vi "testVisa.vi"() -> ()   [LabVIEW 2026]
uses:
  <userlib>/Sensor.ctl
  <vilib>/Instr/_visa.llb/VISA Configure Serial Port (Instr).vi
panel:
  out "Waveform Chart":dbl(graph)
  out "Waveform Graph":waveform(dbl)(graph)
  in  "stop":bool
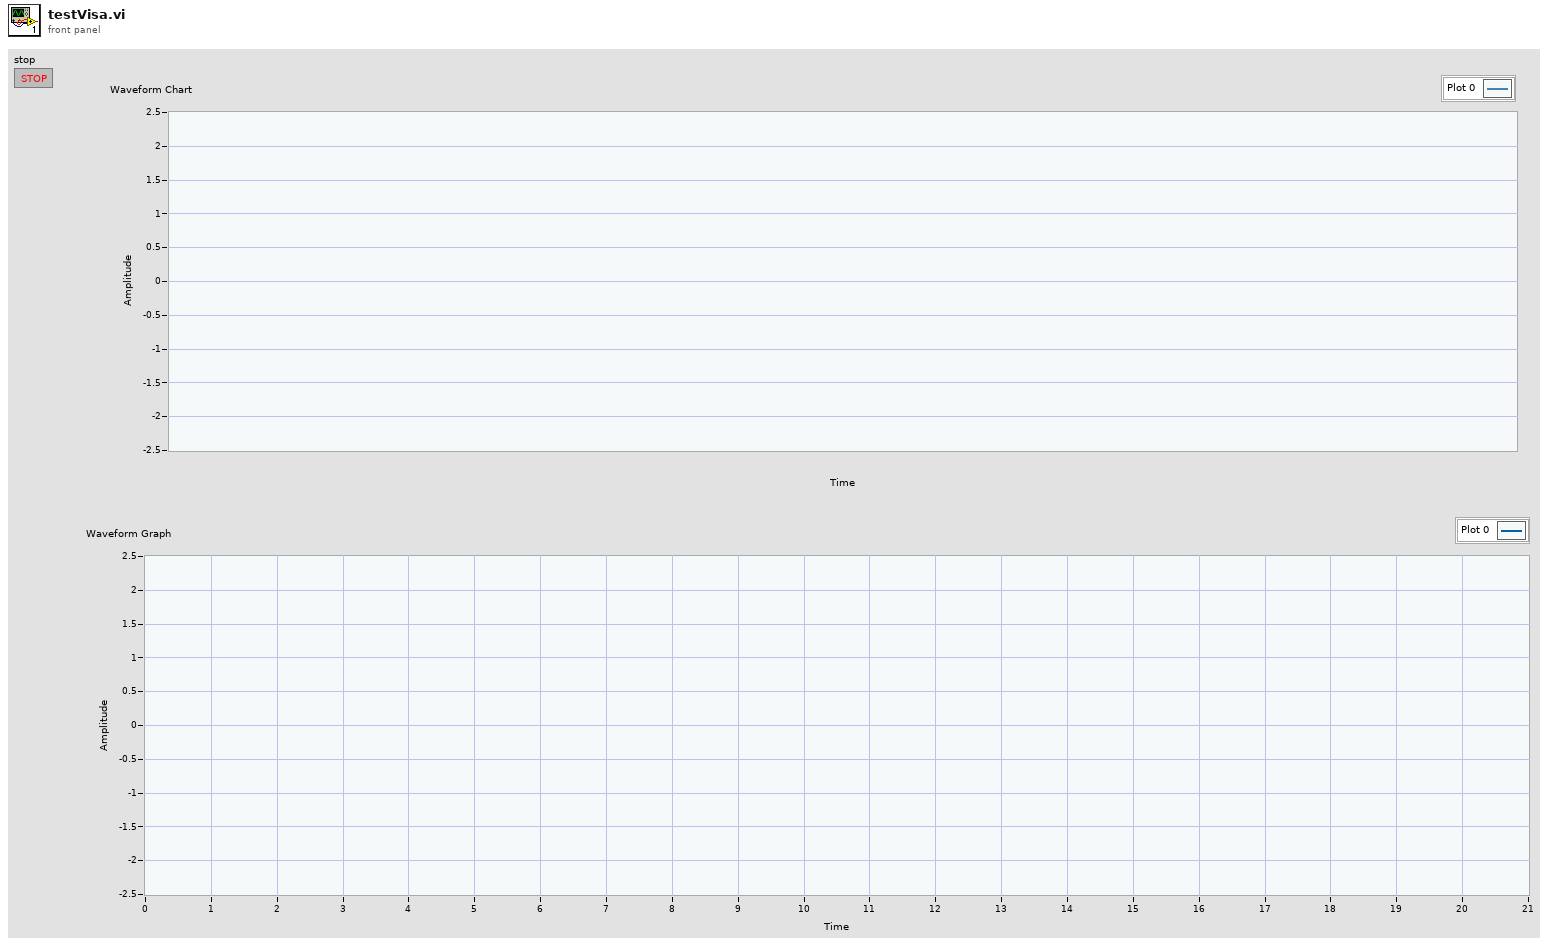
[diagram p1: front panel]
types:
  T1 = typedef "Sensor.ctl" = enum16{"EMG", "ECG", "EEG", "EDA", "ACC", "LUX"}
  T2 = cluster{"Sensor 1":T1, "Sensor 2":T1, "Sensor 3":T1, "Sensor 4":T1, "Sensor 5":T1, "Sensor 6":T1}
  T3 = cluster{"Result":dbl, "Result":dbl, "Result":dbl, "Result":dbl, "Result":dbl, "Result":dbl}
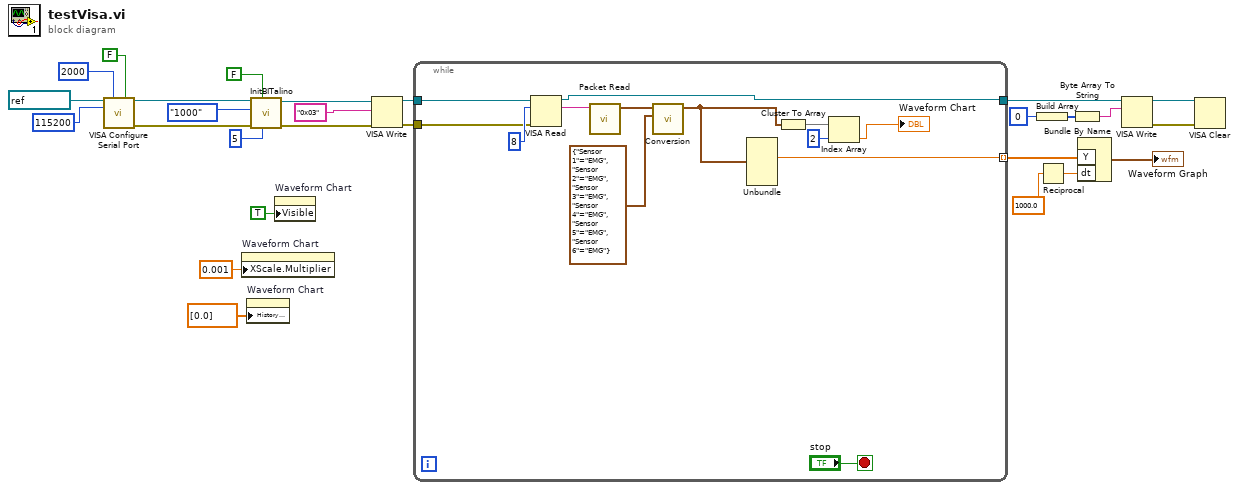
[diagram p0: block diagram]
diagram:
  n1 = call-poly "VISA Configure Serial Port"("VISA resource name"=refnum<visa-resource-name> "COM4", "timeout (10sec)"=u32 2000, "Enable Termination\nChar (T)"=FALSE ("Enable Termination\nChar (T)"), "baud rate (9600)"=u32 115200) -> ("VISA resource name out"=w25:refnum<visa-resource-name>, "error out"=w24:errorcluster)  [unwired: 10 in]
  n2 = property on="Waveform Chart" class="WFChart (strict)"("XScale.Multiplier"=0.001 ("X Scale.Offset and Multiplier:Multiplier")) -> ()  [unwired: 2 in, 2 out]
  n3 = property on="Waveform Chart" class="WFChart (strict)"("History Data"=dbl[] [0.0]) -> ()  [unwired: 2 in, 2 out]
  n4 = call "InitBITalino.vi"("Battery \nThreshold (%)"=u8 5 ("Battery \nThreshold (%)"), "MODE"=FALSE, "error in (no error)"=w24, "Sample Rate"=enum16{"1", "10", "100", "1000"}."1000", "BITalino"=w25) -> ("error out"=w14:errorcluster, "VISA out"=w12:refnum<visa-resource-name>)  [unwired: 4 in, 1 out]
  n5 = property on="Waveform Chart" class="WFChart (strict)"("Visible"=TRUE) -> ()  [unwired: 2 in, 2 out]
  n6 = VISA Write(VISA resource name=w12, write buffer="0x03", error in (no error)=w14) -> (VISA resource name out=w10:refnum<visa-resource-name>, error out=w11:errorcluster)  [unwired: 1 out]
  n7 = while {
    tunnel: [w36] -> w23
    tunnel: w11 -> [w34]
    tunnel: w10 -> [w33]
    tunnel: [w32] -> w5 mode=indexing
    stop <- "stop" stop-if-true
    n8 = VISA Read(VISA resource name=w33, byte count=u32 8, error in (no error)=w34) -> (VISA resource name out=w36:refnum<visa-resource-name>, read buffer=w39:string)  [unwired: 2 out]
    n9 = call "Packet Read.vi"("Packets"=w39) -> ("Analog Channels"=w38:cluster{u16, u16, u16, u16, u16, u16})  [unwired: 7 in, 3 out]
    n10 = call "Conversion.vi"("Sensor Type"=T2 {"Sensor 1"=enum."EMG", "Sensor 2"=enum."EMG", "Sensor 3"=enum."EMG", "Sensor 4"=enum."EMG", "Sensor 5"=enum."EMG", "Sensor 6"=enum."EMG"}, "Analog Channels"=w38) -> ("output cluster"=w31:T3)  [unwired: 8 in, 1 out]
    n11 = Unbundle(w31) -> ("Result"=w32:dbl)  [unwired: 5 out]
    n12 = Cluster To Array(cluster=w31) -> (array=w30:dbl[])
    n13 = Index Array(array=w30, index=2) -> (element=→"Waveform Chart":dbl)
  }
  n14 = Build Array(u8 0) -> (w19:u8[])
  n15 = Reciprocal(x=1000.0) -> (1/x=w9:dbl)
  n16 = Byte Array To String(unsigned byte array=w19) -> (string=w18:string)
  n17 = Bundle By Name("Y"=w5, "dt"=w9) -> (→"Waveform Graph":waveform(dbl))  [unwired: 1 in]
  n18 = VISA Write(VISA resource name=w23, write buffer=w18) -> (VISA resource name out=w22:refnum<visa-resource-name>, error out=w21:errorcluster)  [unwired: 1 in, 1 out]
  n19 = VISA Clear(VISA resource name=w22, error in (no error)=w21) -> ()  [unwired: 2 out]
